vi "Acquire Most Recent Image.vi"() -> ()   [LabVIEW 2019]
doc: "The Acquire Most Recent Image example acquires images continuously and displays the images in an image control using a grab acquisition. It uses the <B>Last New</B> acquisition mode to get the most recent image to avoid waiting for a new image to be acquired."
uses:
  <vilib>/vision/driver/IMAQdx.llb/IMAQdx Buffer Number Mode.ctl
  <vilib>/vision/driver/NI_Vision_Acquisition_Software.lvlib
  <resource>/objmgr/imaqdx.rc
panel:
  in  "ValueDBL":dbl
  out "Acquisition Frame Rate":dbl
  in  "Camera Name":refnum<k21> caption="IMAQdx Session"
  out "Buffer Number":u32
  out "Image":T1(plugin-control)
  in  "Stop":bool
  # "Overview: Demonstrates how to acquire the most recent image continuous from a camer.\nRequirements: Vision Acquisition Software\nInstructions:\n1. Select the Camera Name\n2. Run the VI"
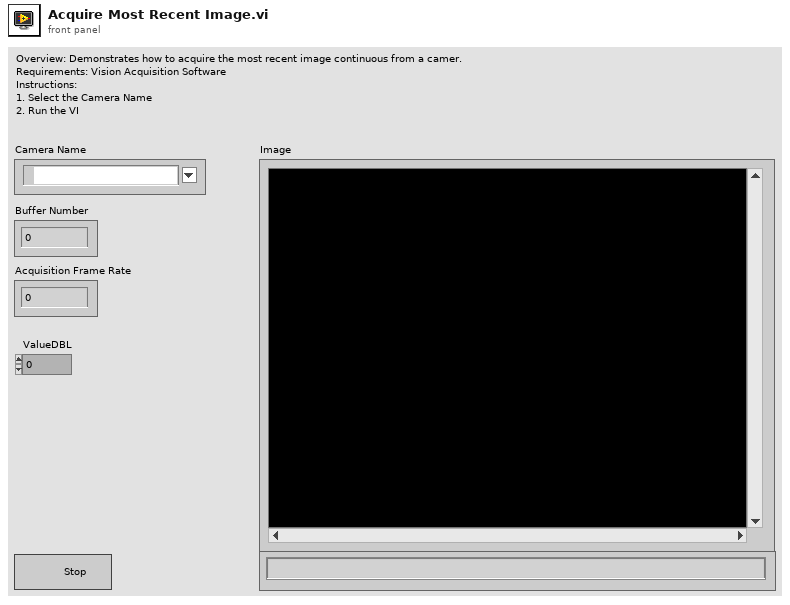
[diagram p1: front panel]
types:
  T1 = typedef "IMAQ Image.ctl" = refnum<image>
  T2 = typedef "IMAQdx.ctl" = refnum<k21>
  T3 = typedef "NI_Vision_Acquisition_Software.lvlib/IMAQdx Buffer Number Mode.ctl" = enum32{"Next", "Last", "Buffer Number", "Every", "Last New"}
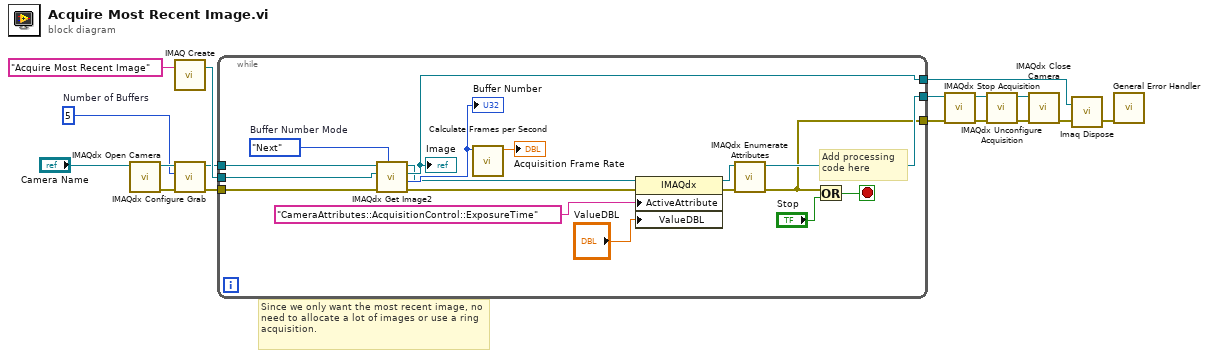
[diagram p0: block diagram]
diagram:
  w4 = u32 5  # Number of Buffers
  # "Since we only want the most recent image, no need to allocate a lot of images or use a ring acquisition."
  n1 = call <vilib>:"IMAQdx Open Camera.vi"("Session In"="Camera Name") -> ("error out"=w3:errorcluster, "Session Out"=w5:T2)  [unwired: 2 in, 7 out]
  n2 = call "IMAQ Create"("Image Name"="Acquire Most Recent Image") -> ("New Image"=w17:T1)  [unwired: 3 in, 2 out]
  n3 = call <vilib>:"IMAQdx Configure Grab.vi"("error in"=w3, "Number of Buffers"=w4, "Session In"=w5) -> ("error out"=w1:errorcluster, "Session Out"=w2:T2)  [unwired: 7 in]
  n4 = while {
    tunnel: [w20] -> w14
    tunnel: w1 -> [w33]
    tunnel: w2 -> [w22]
    tunnel: [w18] -> w15
    tunnel: w17 -> [w32]
    tunnel: [w29] -> w6
    stop <- w34 stop-if-true
    w31 = IMAQdx_Buffer_Number_Mode."Next"  # Buffer Number Mode
    # "Add processing code here"
    n5 = call <vilib>:"IMAQdx Get Image2.vi"("Buffer Number Mode (Next)"=w31, "error in"=w33, "Image In"=w32, "Session In"=w22) -> ("error out"=w19:errorcluster, "Buffer Number Out"=w28:u32, "Image Out"=w29:T1, "Session Out"=w21:T2)  [unwired: 4 in]
    "Image" <- w29
    "Buffer Number" <- w28
    n6 = call <vilib>:"Calculate Frames per Second.vi"("Buffer Number"=w28) -> ("Acquired Frames/s"=→"Acquisition Frame Rate":dbl)  [unwired: 8 in, 2 out]
    n7 = property class="IMAQdx"(reference=w21, error in=w19, "ActiveAttribute"="CameraAttributes::AcquisitionControl::ExposureTime", "ValueDBL"="ValueDBL") -> (reference out=w24:T2, error out=w23:errorcluster)
    n8 = call <vilib>:"IMAQdx Enumerate Attributes.vi"("error in"=w23, "Session In"=w24) -> ("error out"=w18:errorcluster, "Session Out"=w20:T2)  [unwired: 7 in, 1 out]
    n9 = Or(x=w18, y="Stop") -> (x .or. y?=w34:bool)
  }
  n10 = call <vilib>:"IMAQdx Stop Acquisition.vi"("error in"=w15, "Session In"=w14) -> ("error out"=w10:errorcluster, "Session Out"=w11:T2)  [unwired: 8 out]
  n11 = call <vilib>:"IMAQdx Unconfigure Acquisition.vi"("error in"=w10, "Session In"=w11) -> ("error out"=w13:errorcluster, "Session Out"=w12:T2)  [unwired: 8 out]
  n12 = call <vilib>:"IMAQdx Close Camera.vi"("error in"=w13, "Session In"=w12) -> ("error out"=w9:errorcluster)  [unwired: 9 out]
  n13 = call "Imaq Dispose"("Image"=w6, "error in (no error)"=w9) -> ("error out"=w8:errorcluster)  [unwired: 4 in]
  n14 = call <vilib>:"General Error Handler.vi"("error in (no error)"=w8) -> ()  [unwired: 2 in, 13 out]
